vi "Read MsgReceived.vi"(8 "error in (no error)":errorcluster, 11 "TCPComEvents in":refnum<class "TCPComEvents.lvclass">) -> (0 "error out":errorcluster, 2 "MsgReceived":refnum<user-event>, 3 "TCPComEvents out":refnum<class "TCPComEvents.lvclass">)   [LabVIEW 2016, in "TCPComEvents.lvclass"]
uses:
  TCPComEvents.lvclass
  TCPComEvents.lvclass/TCPComEvents.ctl
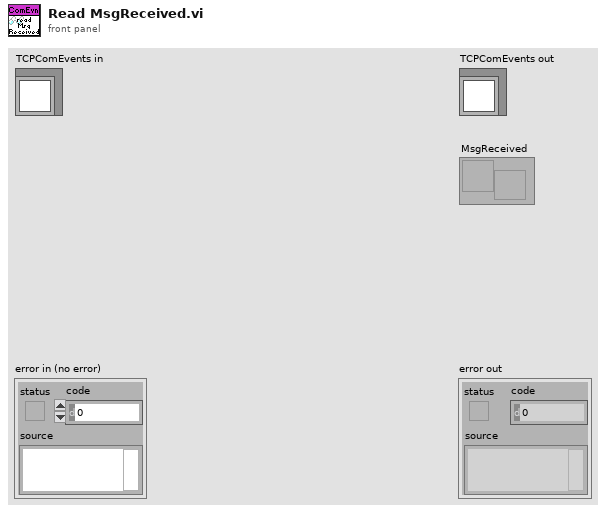
[diagram p1: front panel]
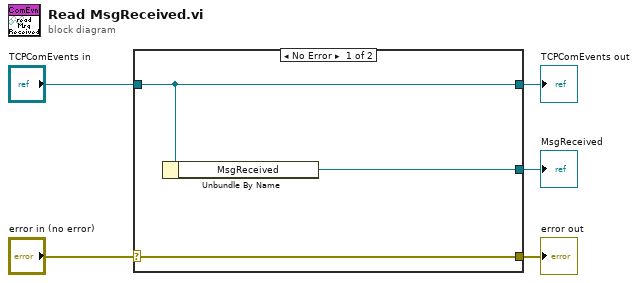
[diagram p0: block diagram]
diagram:
  n1 = case shown="No Error" "error in (no error)" {
    selector: "error in (no error)" -> [w8 w9]
    tunnel: [w8 w9] -> w4
    tunnel: [w7 w10] -> w2
    tunnel: "TCPComEvents in" -> [w7 w10]
    tunnel: [w6 _] -> w1
    frame No Error {
      n2 = Unbundle By Name(w7) -> ("MsgReceived"=w6:refnum<user-event>)
    }
    frame Error {
    }
  }
  "error out" <- w4
  "TCPComEvents out" <- w2
  "MsgReceived" <- w1
